vi "Example.vi"() -> ()   [LabVIEW 2016, in "pl1000.lvlib"]
uses:
  pl1000.lvlib
panel:
  out "Ready":bool=TRUE
  out "overflow":bool[](array[boolean])=[FALSE, FALSE, FALSE, FALSE, FALSE, FALSE, TRUE, FALSE, FALSE, FALSE, FALSE, FALSE, FALSE, FALSE, FALSE, FALSE]
  out "Waveform Chart":dbl[](graph)=[0.0, 0.0, 0.0, 0.0, 0.0, 0.0, 0.0, 0.0, 0.0, 0.0, 0.0, 0.0, 0.0, 0.0, 0.0, 0.0, 0.0, 0.0, 0.0, 0.0, 0.0, 0.0, 0.0, 0.0, 0.0, 0.0, 0.0, 0.0, 0.0, 0.0, 0.0, 0.0, 0.0, 0.0, 0.0, 0.0, 0.0, 0.0, 0.0, 0.0, 0.0, 0.0, 0.0, 0.0, 0.0006105006105006105, 0.0, 0.0, 0.0006105006105006105, 0.0, 0.0, 0.0, 0.0006105006105006105, 0.0, 0.0, 0.0, 0.0, 0.0, 0.0, 0.0, 0.0, 0.0, 0.0, 0.0, 0.0, 0.0, 0.0, 0.0, 0.0, 0.0, 0.0, 0.0, 0.0, 0.0, 0.0, 0.0006105006105006105, 0.0, 0.0, 0.0, 0.0006105006105006105, 0.0, 0.0006105006105006105, 0.0, 0.0, 0.0006105006105006105, 0.0, 0.0, 0.0, 0.0, 0.0, 0.0, 0.0, 0.0, 0.0, 0.0, 0.0, 0.0, 0.0, 0.0, 0.0, 0.0, 0.0, 0.0, 0.0, 0.0, 0.0006105006105006105, 0.0, 0.0, 0.0, 0.0006105006105006105, 0.0, 0.0, 0.0, 0.0, 0.0, 0.0, 0.0, 0.0, 0.0, 0.0, 0.0, 0.0, 0.0, 0.0, 0.0, 0.0, 0.0, 0.0, 0.0, 0.0, 0.0, 0.0, 0.0, 0.0, 0.0, 0.0, 0.0, 0.0, 0.0, 0.0, 0.0, 0.0, 0.0006105006105006105, 0.0, 0.0, 0.0006105006105006105, 0.0, 0.0, 0.0, 0.0, 0.0, 0.0, 0.0, 0.0, 0.0, 0.0, 0.0, 0.0, 0.0, 0.0, 0.0, 0.0006105006105006105, 0.0, 0.0, 0.0, 0.0, 0.0, 0.0, 0.0, 0.0, 0.0, 0.0, 0.0, 0.0, 0.0, 0.0, 0.0, 0.0, 0.0, 0.0, 0.0, 0.0, 0.0, 0.0, 0.0, 0.0, 0.0, 0.0, 0.0, 0.0, 0.0, 0.0, 0.0, 0.0, 0.0, 0.0, 0.0, 0.0, 0.0, 0.0, 0.0, 0.0, 0.0, 0.0, 0.0, 0.0, 0.0006105006105006105, 0.0, 0.0, 0.0, 0.0, 0.0, 0.0, 0.0, 0.0, 0.0, 0.0, 0.0, 0.0, 0.0, 0.0, 0.0, 0.0, 0.0, 0.0, 0.0, 0.0, 0.0, 0.0, 0.0, 0.0, 0.0, 0.0006105006105006105, 0.0, 0.0, 0.0, 0.0, 0.0, 0.0, 0.0, 0.0, 0.0, 0.0, 0.0, 0.0, 0.0, 0.0, 0.0, 0.0, 0.0, 0.0, 0.0, 0.0, 0.0, 0.0, 0.0, 0.0, 0.0, 0.0, 0.0, 0.0, 0.0, 0.0, 0.0, 0.0, 0.0, 0.0, 0.0, 0.0, 0.0, 0.0, 0.0, 0.0, 0.0, 0.0, 0.0, 0.0, 0.0, 0.0, 0.0, 0.0, 0.0, 0.0, 0.0, 0.0, 0.0, 0.0, 0.0, 0.0, 0.0, 0.0, 0.0, 0.0, 0.0, 0.0, 0.0, 0.0, 0.0, 0.0, 0.0, 0.0, 0.0, 0.0, 0.0, 0.0, 0.0, 0.0, 0.0, 0.0, 0.0, 0.0, 0.0006105006105006105, 0.0, 0.0, 0.0, 0.0, 0.0, 0.0, 0.0, 0.0, 0.0, 0.0, 0.0, 0.0, 0.0, 0.0, 0.0, 0.0, 0.0, 0.0, 0.0, 0.0, 0.0, 0.0, 0.0, 0.0, 0.0, 0.0, 0.0, 0.0, 0.0, 0.0, 0.0, 0.0, 0.0, 0.0, 0.0, 0.0, 0.0, 0.0, 0.0, 0.0, 0.0, 0.0, 0.0, 0.0, 0.0, 0.0, 0.0, 0.0, 0.0, 0.0, 0.0, 0.0, 0.0, 0.0, 0.0, 0.0, 0.0, 0.0, 0.0, 0.0, 0.0, 0.0, 0.0, 0.0, 0.0, 0.0, 0.0, 0.0, 0.0, 0.0, 0.0, 0.0, 0.0, 0.0, 0.0, 0.0, 0.0, 0.0, 0.0, 0.0, 0.0, 0.0, 0.0, 0.0, 0.0, 0.0, 0.0, 0.0, 0.0, 0.0, 0.0, 0.0, 0.0, 0.0, 0.0, 0.0006105006105006105, 0.0, 0.0, 0.0, 0.0006105006105006105, 0.0, 0.0, 0.0, 0.0, 0.0, 0.0, 0.0, 0.0, 0.0, 0.0, 0.0, 0.0, 0.0, 0.0, 0.0, 0.0, 0.0, 0.0, 0.0, 0.0, 0.0, 0.0, 0.0, 0.0, 0.0, 0.0, 0.0, 0.0, 0.0, 0.0, 0.0, 0.0006105006105006105, 0.0, 0.0, 0.0, 0.0, 0.0, 0.0, 0.0, 0.0, 0.0, 0.0, 0.0, 0.0, 0.0, 0.0, 0.0006105006105006105, 0.0, 0.0, 0.0, 0.0, 0.0, 0.0, 0.0006105006105006105, 0.0, 0.0, 0.0, 0.0, 0.0006105006105006105, 0.0, 0.0, 0.0, 0.0, 0.0, 0.0, 0.0, 0.0, 0.0, 0.0, 0.0006105006105006105, 0.0, 0.0, 0.0, 0.0, 0.0, 0.0, 0.0, 0.0, 0.0, 0.0, 0.0, 0.0, 0.0, 0.0, 0.0, 0.0, 0.0, 0.0, 0.0, 0.0006105006105006105, 0.0, 0.0, 0.0, 0.0, 0.0, 0.0, 0.0, 0.0, 0.0, 0.0, 0.0, 0.0, 0.0, 0.0, 0.0, 0.0, 0.0, 0.0, 0.0, 0.0, 0.0, 0.0, 0.0, 0.0006105006105006105, 0.0, 0.0006105006105006105, 0.0, 0.0, 0.0, 0.0006105006105006105, 0.0, 0.0, 0.0, 0.0, 0.0, 0.0, 0.0, 0.0, 0.0, 0.0, 0.0006105006105006105, 0.0, 0.0, 0.0, 0.0, 0.0, 0.0, 0.0, 0.0, 0.0, 0.0, 0.0, 0.0, 0.0, 0.0, 0.0, 0.0006105006105006105, 0.0, 0.0, 0.0, 0.0, 0.0, 0.0, 0.0006105006105006105, 0.0, 0.0, 0.0, 0.0, 0.0006105006105006105, 0.0, 0.0, 0.0, 0.0, 0.0, 0.0, 0.0, 0.0, 0.0, 0.0, 0.0, 0.0006105006105006105, 0.0, 0.0, 0.0, 0.0, 0.0, 0.0006105006105006105, 0.0, 0.0, 0.0, 0.0, 0.0, 0.0, 0.0006105006105006105, 0.0006105006105006105, 0.0, 0.0, 0.0, 0.0, 0.0, 0.0, 0.0, 0.0, 0.0, 0.0, 0.0, 0.0, 0.0, 0.0, 0.0, 0.0, 0.0, 0.0, 0.0, 0.0, 0.0, 0.0, 0.0, 0.0, 0.0, 0.0, 0.0, 0.0, 0.0, 0.0, 0.0006105006105006105, 0.0, 0.0, 0.0, 0.0, 0.0, 0.0, 0.0, 0.0, 0.0, 0.0, 0.0, 0.0, 0.0, 0.0, 0.0, 0.0, 0.0, 0.0, 0.0, 0.0, 0.0, 0.0, 0.0, 0.0, 0.0, 0.0, 0.0, 0.0006105006105006105, 0.0, 0.0, 0.0, 0.0, 0.0, 0.0, 0.0, 0.0, 0.0, 0.0, 0.0, 0.0, 0.0, 0.0, 0.0, 0.0, 0.0, 0.0, 0.0, 0.0, 0.0, 0.0, 0.0, 0.0, 0.0, 0.0, 0.0, 0.0, 0.0, 0.0, 0.0, 0.0, 0.0, 0.0, 0.0, 0.0, 0.0, 0.0, 0.0, 0.0, 0.0, 0.0, 0.0006105006105006105, 0.0006105006105006105, 0.0, 0.0, 0.0, 0.0, 0.0, 0.0, 0.0, 0.0, 0.0, 0.0, 0.0, 0.0006105006105006105, 0.0, 0.0, 0.0, 0.0, 0.0, 0.0, 0.0, 0.0006105006105006105, 0.0, 0.0, 0.0, 0.0, 0.0, 0.0006105006105006105, 0.0, 0.0006105006105006105, 0.0, 0.0, 0.0, 0.0, 0.0, 0.0, 0.0, 0.0, 0.0, 0.0, 0.0, 0.0, 0.0, 0.0, 0.0, 0.0, 0.0, 0.0, 0.0, 0.0, 0.0006105006105006105, 0.0, 0.0, 0.0, 0.0, 0.0006105006105006105, 0.0, 0.0, 0.0, 0.0, 0.0, 0.0, 0.0, 0.0, 0.0, 0.0, 0.0, 0.0, 0.0, 0.0, 0.0, 0.0, 0.0, 0.0, 0.0, 0.0, 0.0, 0.0, 0.0, 0.0, 0.0, 0.0, 0.0, 0.0, 0.0, 0.0, 0.0, 0.0, 0.0, 0.0, 0.0, 0.0, 0.0006105006105006105, 0.0, 0.0, 0.0, 0.0, 0.0, 0.0, 0.0, 0.0, 0.0, 0.0, 0.0, 0.0, 0.0, 0.0006105006105006105, 0.0, 0.0, 0.0, 0.0, 0.0, 0.0, 0.0, 0.0, 0.0, 0.0, 0.0, 0.0, 0.0, 0.0, 0.0, 0.0, 0.0, 0.0, 0.0, 0.0, 0.0, 0.0, 0.0, 0.0, 0.0, 0.0, 0.0, 0.0, 0.0, 0.0, 0.0, 0.0, 0.0, 0.0, 0.0, 0.0, 0.0, 0.0, 0.0, 0.0, 0.0, 0.0, 0.0, 0.0, 0.0, 0.0, 0.0, 0.0, 0.0, 0.0, 0.0, 0.0006105006105006105, 0.0, 0.0, 0.0, 0.0, 0.0, 0.0, 0.0, 0.0, 0.0, 0.0, 0.0, 0.0, 0.0, 0.0, 0.0, 0.0, 0.0, 0.0, 0.0, 0.0, 0.0, 0.0, 0.0, 0.0, 0.0, 0.0, 0.0, 0.0, 0.0, 0.0, 0.0, 0.0, 0.0006105006105006105, 0.0, 0.0006105006105006105, 0.0, 0.0, 0.0, 0.0, 0.0, 0.0, 0.0, 0.0006105006105006105, 0.0, 0.0, 0.0, 0.0, 0.0, 0.0, 0.0, 0.0, 0.0, 0.0, 0.0, 0.0, 0.0, 0.0, 0.0, 0.0, 0.0, 0.0, 0.0, 0.0, 0.0, 0.0, 0.0, 0.0, 0.0, 0.0006105006105006105, 0.0, 0.0, 0.0, 0.0, 0.0, 0.0, 0.0, 0.0, 0.0, 0.0, 0.0, 0.0, 0.0, 0.0, 0.0, 0.0, 0.0, 0.0, 0.0, 0.0006105006105006105, 0.0, 0.0, 0.0, 0.0, 0.0, 0.0, 0.0, 0.0, 0.0, 0.0, 0.0, 0.0, 0.0, 0.0, 0.0, 0.0, 0.0, 0.0, 0.0, 0.0, 0.0, 0.0, 0.0, 0.0, 0.0, 0.0, 0.0, 0.0, 0.0, 0.0, 0.0, 0.0, 0.0, 0.0, 0.0, 0.0, 0.0, 0.0, 0.0, 0.0, 0.0, 0.0, 0.0, 0.0, 0.0, 0.0, 0.0, 0.0, 0.0, 0.0, 0.0, 0.0, 0.0, 0.0, 0.0]
  out "Unit Info":string="PICO_DRIVER_VERSION  :      2.0.17.1457 \r\nPICO_USB_VERSION :      USB 1.1 \r\nPICO_HARDWARE_VERSION :      1 \r\nPICO_VARIANT_INFO :      PicoLog1216 \r\nPICO_BATCH_AND_SERIAL  :      GW077/175 \r\nPICO_CAL_DATE :      12Apr19 \r\nPICO_KERNEL_VERSION :      PICOPP.SYS V1.0 \r\n"
  out "Open progress":u8(slide) scale=0.0..100.0
  in  "Async Open":bool
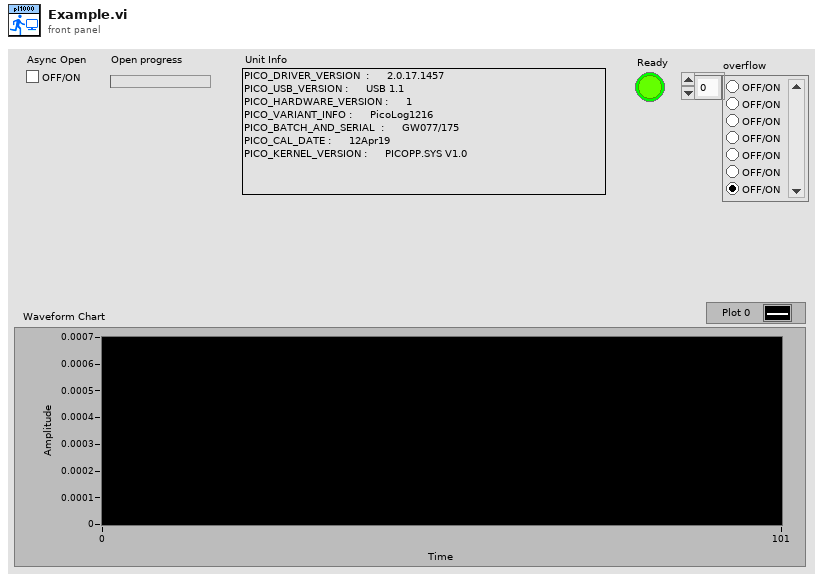
[diagram p1: front panel]
types:
  T1 = enum32{"PICO_DRIVER_VERSION ", "PICO_USB_VERSION", "PICO_HARDWARE_VERSION", "PICO_VARIANT_INFO", "PICO_BATCH_AND_SERIAL ", "PICO_CAL_DATE", "PICO_KERNEL_VERSION"}[]
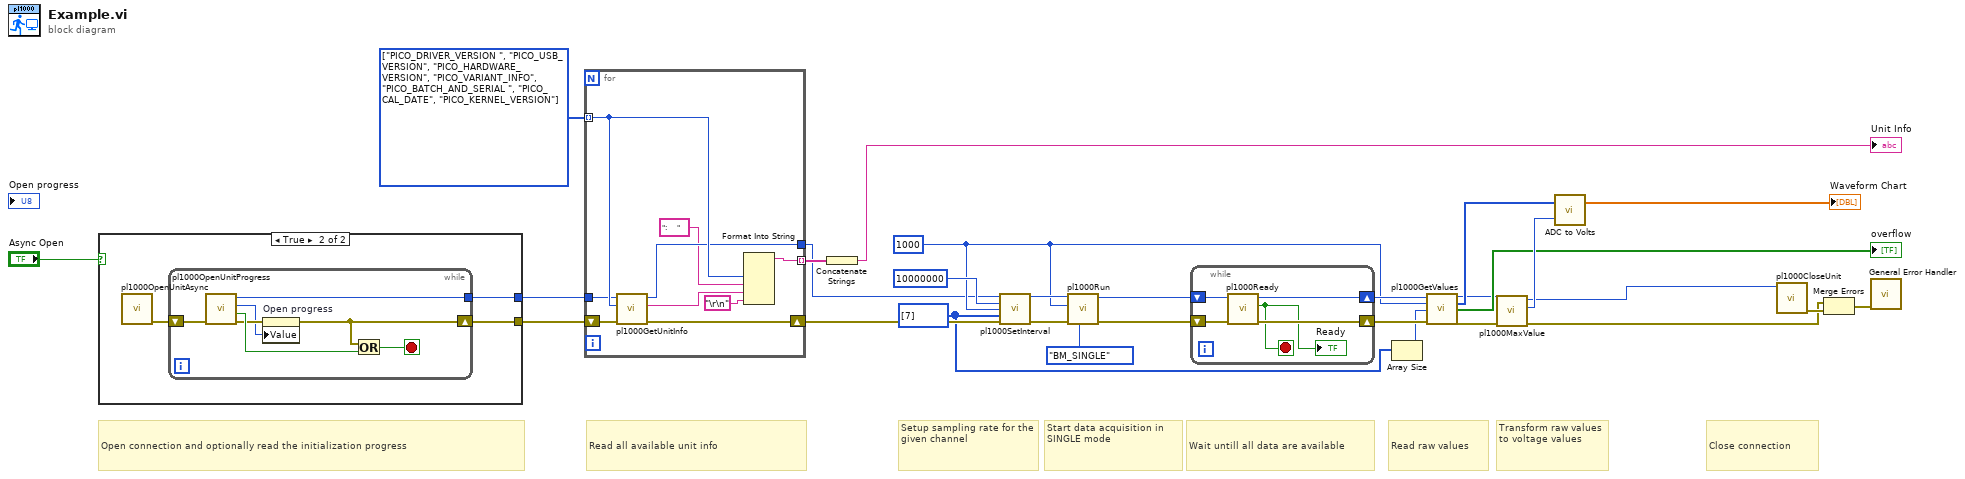
[diagram p0: block diagram]
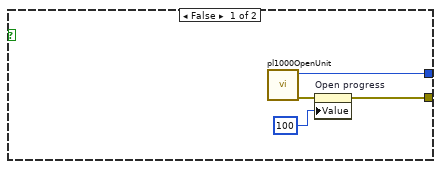
[diagram p2: hidden frame]
diagram:
  w2 = i16[] [7] ("channels")
  w9 = u32 1000 ("idealNoOfSamples")
  w28 = T1 [enum."PICO_DRIVER_VERSION ", enum."PICO_USB_VERSION", enum."PICO_HARDWARE_VERSION", enum."PICO_VARIANT_INFO", enum."PICO_BATCH_AND_SERIAL ", enum."PICO_CAL_DATE", enum."PICO_KERNEL_VERSION"] items=["PICO_DRIVER_VERSION ", "PICO_USB_VERSION", "PICO_HARDWARE_VERSION", "PICO_VARIANT_INFO", "PICO_BATCH_AND_SERIAL ", "PICO_CAL_DATE", "PICO_KERNEL_VERSION"] ("Info")
  # "Close connection"
  # "Transform raw values to voltage values"
  # "Read raw values"
  # "Wait untill all data are available"
  # "Start data acquisition in SINGLE mode"
  # "Setup sampling rate for the given channel"
  # "Read all available unit info"
  # "Open connection and optionally read the initialization progress"
  n1 = case shown="True" "Async Open" {
    tunnel: [w31 w34] -> w26
    tunnel: [w33 w35] -> w27
    frame False {
      n2 = call "pl1000OpenUnit.vi"() -> ("error out"=w32:errorcluster, "pl1000 handle out"=w33:i16)  [unwired: 10 in]
      n3 = property on="Open progress" class="Slide (strict)"(error in=w32, "Value"=u8 100 ("Open progress")) -> (error out=w31:errorcluster)  [unwired: 1 in, 1 out]
    }
    frame True {
      n4 = call "pl1000OpenUnitAsync.vi"() -> ("error out"=w36:errorcluster)  [unwired: 10 in, 1 out]
      n5 = while {
        shift-right: [w37] -> w34
        shift-left: w36 -> [w42]
        tunnel: [w41] -> w35
        stop <- w38 stop-if-true
        n6 = call "pl1000OpenUnitProgress.vi"("error in (no error)"=w42) -> ("error out"=w40:errorcluster, "complete"=w43:bool, "progress"=w39:i32, "pl1000 handle out"=w41:i16)  [unwired: 7 in]
        n7 = property on="Open progress" class="Slide (strict)"(error in=w40, "Value"=w39) -> (error out=w37:errorcluster)  [unwired: 1 in, 1 out]
        n8 = Or(x=w37, y=w43) -> (x .or. y?=w38:bool)
      }
    }
  }
  n9 = for {
    tunnel: w28 -> [w52] mode=indexing
    tunnel: w27 -> [w51]
    shift-right: [w49] -> w4
    shift-left: w26 -> [w50]
    tunnel: [w48] -> w5
    tunnel: [w47] -> w25 mode=indexing
    n10 = call "pl1000GetUnitInfo.vi"("error in (no error)"=w50, "Info"=w52, "pl1000 handle"=w51) -> ("error out"=w49:errorcluster, "String"=w44:string, "pl1000 handle out"=w48:i16)  [unwired: 6 in]
    n11 = Format Into String(w52, ":     " ("input 3"), w44, "\r\n") -> (resulting string=w47:string)  [unwired: 3 in, 1 out]
  }
  n12 = Concatenate Strings(w25) -> (→"Unit Info":string)
  n13 = call "pl1000SetInterval.vi"("pl1000 handle"=w5, "usForBlock"=u32 10000000, "idealNoOfSamples"=w9, "channels"=w2, "error in (no error)"=w4) -> ("pl1000 handle out"=w15:i16, "error out"=w14:errorcluster)  [unwired: 9 in]
  n14 = call "pl1000Run.vi"("method"=enum16{"BM_SINGLE", "BM_WINDOW", "BM_STREAM"}."BM_SINGLE", "error in (no error)"=w14, "noOfValues"=w9, "pl1000 handle"=w15) -> ("error out"=w18:errorcluster, "pl1000 handle out"=w19:i16)  [unwired: 6 in]
  n15 = while {
    shift-right: [w55] -> w17
    shift-left: w19 -> [w57]
    shift-right: [w54] -> w16
    shift-left: w18 -> [w56]
    stop <- w53 stop-if-true
    n16 = call "pl1000Ready.vi"("error in (no error)"=w56, "pl1000 handle"=w57) -> ("error out"=w54:errorcluster, "ready"=w53:bool, "pl1000 handle out"=w55:i16)  [unwired: 7 in]
    "Ready" <- w53
  }
  n17 = Array Size(array=w2) -> (size(s)=w1:i32)
  n18 = call "pl1000GetValues.vi"("pl1000 handle"=w17, "noOfValues"=w9, "nOfChannels"=w1, "error in (no error)"=w16) -> ("pl1000 handle out"=w7:i16, "values"=w12:u16[], "overflow"=→"overflow":bool[], "error out"=w8:errorcluster)  [unwired: 6 in, 2 out]
  n19 = call "pl1000MaxValue.vi"("error in (no error)"=w8, "pl1000 handle"=w7) -> ("error out"=w3:errorcluster, "maxValue"=w13:u16, "pl1000 handle out"=w6:i16)  [unwired: 7 in]
  n20 = call "ADC to Volts.vi"("maxValue"=w13, "ADC values"=w12) -> ("values in Volt"=→"Waveform Chart":dbl[])  [unwired: 1 in]
  n21 = call "pl1000CloseUnit.vi"("pl1000 handle"=w6) -> ("error out"=w22:errorcluster)  [unwired: 9 in, 1 out]
  n22 = Merge Errors(w3, w22) -> (w21:errorcluster)
  n23 = call <vilib>:"General Error Handler.vi"("error in (no error)"=w21) -> ()  [unwired: 10 in, 5 out]
